vi "OnLoad - Remove CD Ports Wihout Referenced NI-XNET Port.vi"(8 "error in (no error)":errorcluster, 10 "Force Delete (F)":bool, 11 "Device Item Ref in in":T1 format="%.0x") -> (0 "error out":errorcluster, 3 "Device Item Ref out":T1 format="%.0x")   [LabVIEW 2017, in "NI-XNET Monitor System Explorer.lvlib"]
uses:
  NI-XNET Monitor System Explorer.lvlib
  <vilib>/NI Veristand/Custom Device API/Custom Device Item Ref.ctl
  <vilib>/NI Veristand/Custom Device API/Custom Device API.lvlib
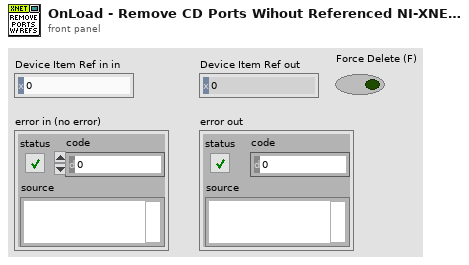
[diagram p1: front panel]
types:
  T1 = typedef "Custom Device API.lvlib/Custom Device Item Ref.ctl" = u64
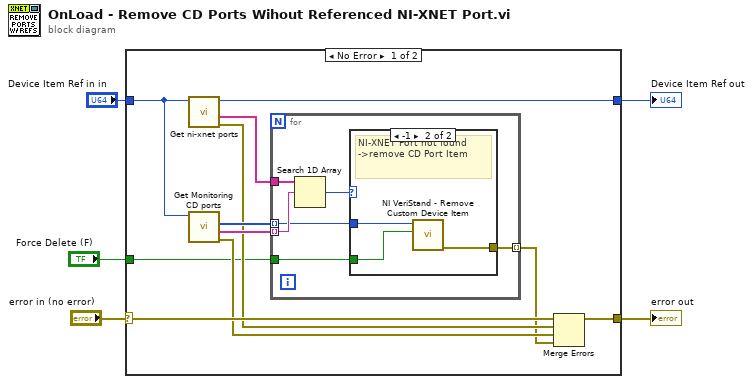
[diagram p0: block diagram]
diagram:
  n1 = case shown="No Error" "error in (no error)" {
    selector: "error in (no error)" -> [w16 w27]
    tunnel: [w8 w27] -> w3
    tunnel: "Device Item Ref in in" -> [w15 w26]
    tunnel: [w14 w26] -> w5
    tunnel: "Force Delete (F)" -> [w6 _]
    frame No Error {
      n2 = call "Get ni-xnet ports.vi"("Device Item Ref in"=w15) -> ("Error Out"=w10:errorcluster, "NI-XNET Port Item Paths"=w11:string[], "Device Item Ref out"=w14:T1)  [unwired: 7 in, 1 out]
      n3 = call "Get Monitoring CD ports.vi"("Device Item Ref in"=w15) -> ("Error Out"=w9:errorcluster, "Referenced NI-XNET Port Item Paths"=w13:string[], "CD Port Refs"=w12:T1[])  [unwired: 7 in, 1 out]
      n4 = for {
        tunnel: w13 -> [w21] mode=indexing
        tunnel: w12 -> [w19] mode=indexing
        tunnel: w11 -> [w22]
        tunnel: [w18] -> w7 mode=indexing
        tunnel: w6 -> [w17]
        n5 = Search 1D Array(1D array=w22, element=w21) -> (index of element=w20:i32)  [unwired: 1 in]
        n6 = case shown="-1" w20 {
          tunnel: w19 -> [_ w25]
          tunnel: [_ w24] -> w18
          tunnel: w17 -> [_ w23]
          frame Default {
            # "Port found do nothing"
          }
          frame -1 {
            # "NI-XNET Port not found ->remove CD Port Item"
            n7 = call <vilib>:"NI VeriStand - Remove Custom Device Item.vi"("Force Delete (F)"=w23, "Item Ref in"=w25) -> ("error out"=w24:errorcluster)  [unwired: 8 in, 1 out]
          }
        }
      }
      n8 = Merge Errors(w16, w10, w9, w7) -> (w8:errorcluster)
    }
    frame Error {
    }
  }
  "Device Item Ref out" <- w5
  "error out" <- w3
